vi "Geometric Match2.vi"(0 "Template File Path":path=path "C:/Users/Admin/Desktop/Main_Module_Assembly/Pattern recognition/templates/color.png", 1 "Image Src":T1, 2 "error in (no error)":errorcluster, 3 "Minimum Match Score":sgl=800.0) -> (4 "Score":dbl, 5 "x rel move":dbl, 6 "y rel move":dbl, 7 "Matched?":bool, 8 "error out":errorcluster)   [LabVIEW 2011]
uses:
  <vilib>/vision/Pattern Matching.llb/IMAQ GM Match Report.ctl
  <vilib>/vision/Image Controls.llb/IMAQ Image.ctl
  <vilib>/vision/NI_Vision_Development_Module.lvlib
panel:
  in  "Scale Factor":sgl=0.000429
  out "y":sgl
  out "x":sgl
  in  "ROI Descriptor":T2 {"Contours"."Type" items=["No Selection", "Point", "Line", "Rectangle", "Oval", "Polygon", "Freehand Region", "Annulus", "Unused2", "Unused3", "Broken Line", "Freehand Line", "Rotated Rectangle"]}
  in  "Color Plane":i32(ring)=5 items=["Red", "Green", "Blue", "Hue", "Saturation", "Luminance", "Value", "Intensity"]
  out "Image Out":T1(plugin-control)
  out "Calibrated Matches (Geometric Matching 1)":T3[](array[typedef]) {"Correlation Score" format="%.2f"; "Target Template Curve Score" format="%.2f"; "Template Target Curve Score" format="%.2f"; "Bounding Box"."y" format="%.2f"; "Bounding Box"."x" format="%.2f"; "Position"."y" format="%.2f"; "Position"."x" format="%.2f"; "Score" format="%.2f"; "Scale" format="%.2f"; "Angle" format="%.2f"; "Occlusion %" format="%.2f"}
  out "Number of Matches (Geometric Matching 1)":i32
  out "Matches (Geometric Matching 1)":T3[](array[typedef]) {"Correlation Score" format="%.2f"; "Target Template Curve Score" format="%.2f"; "Template Target Curve Score" format="%.2f"; "Bounding Box"."y" format="%.2f"; "Bounding Box"."x" format="%.2f"; "Position"."y" format="%.2f"; "Position"."x" format="%.2f"; "Score" format="%.2f"; "Scale" format="%.2f"; "Angle" format="%.2f"; "Occlusion %" format="%.2f"}
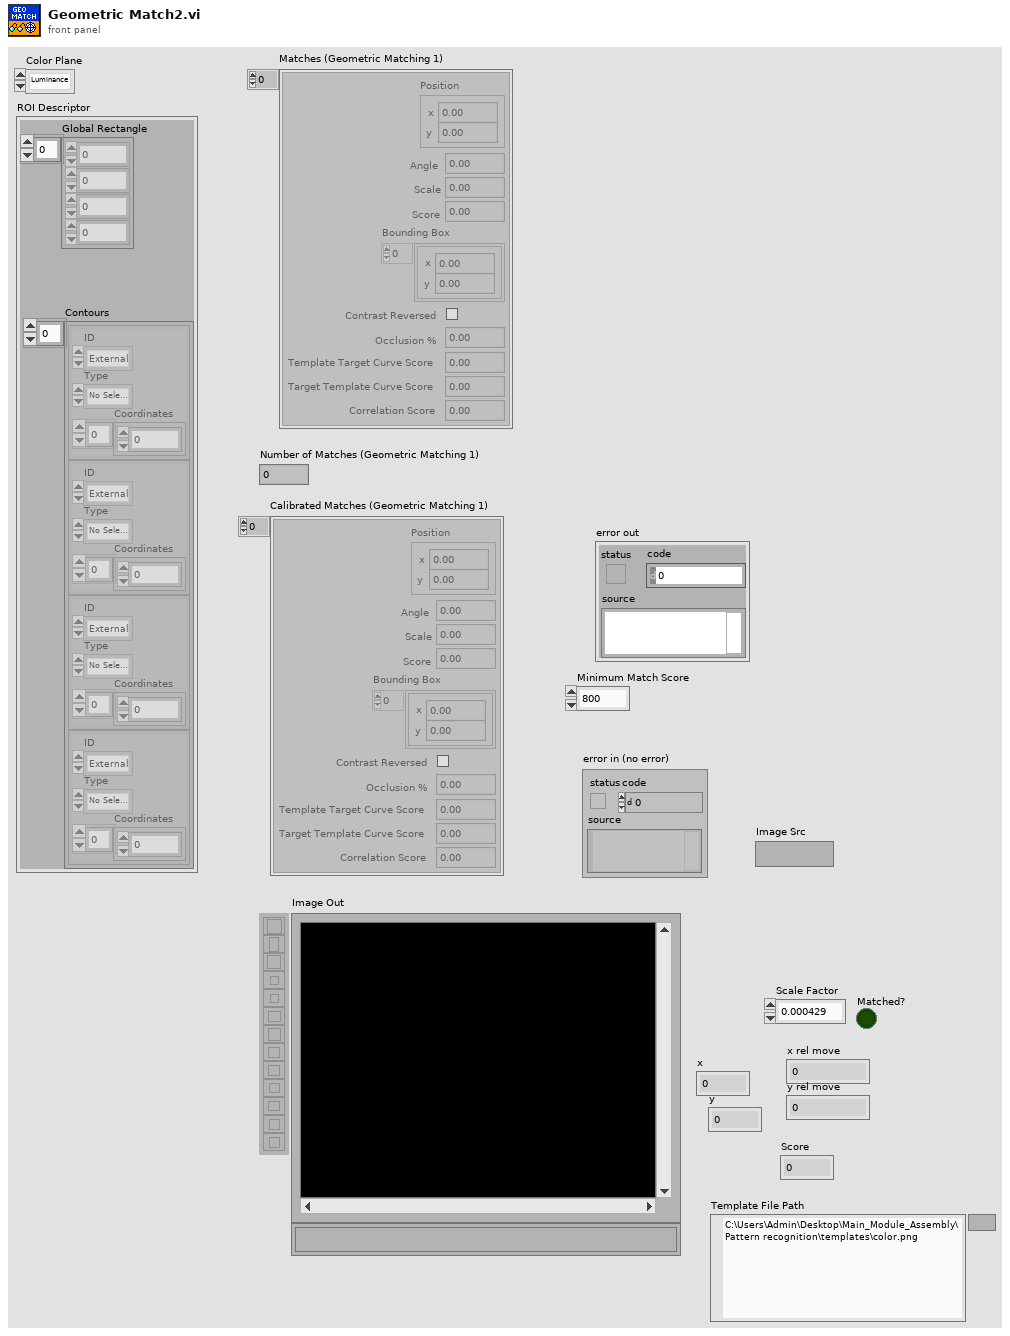
[diagram p1: front panel]
types:
  T1 = typedef "IMAQ Image.ctl" = refnum<image>
  T2 = cluster{"Global Rectangle":i32[], "Contours":cluster{"ID":enum32{"External", "Internal"}, "Type":u32, "Coordinates":i32[]}[]}
  T3 = typedef "IMAQ GM Match Report.ctl" = cluster{"Position":cluster{"x":sgl, "y":sgl}, "Angle":sgl, "Scale":sgl, "Score":sgl, "Bounding Box":cluster{"x":sgl, "y":sgl}[], "Contrast Reversed":bool, "Occlusion %":sgl, "Template Target Curve Score":sgl, "Target Template Curve Score":sgl, "Correlation Score":sgl}
  T4 = cluster{"Setup Data Item":u16, "Item Value":dbl}[]
  T5 = cluster{"Match Constraints":u32, "Min":dbl, "Max":dbl}[]
  T6 = cluster{"Rotation":bool, "Scale":bool, "Occlusion":bool, "Reserved":bool, "Reserved":bool, "Reserved":bool}
  T7 = cluster{"Extraction Mode":u32, "Edge Threshold":i32, "Edge Filter Size":u32, "Min Length":i32, "Row Search Step Size":i32, "Col Search Step Size":i32, "Max Endpoint Gap":i32, "Closed":bool, "Subpixel":bool}
  T8 = cluster{"Curve Parameters":cluster{"Extraction Mode":u32, "Edge Threshold":i32, "Edge Filter Size":u32, "Min Length":i32, "Row Search Step Size":i32, "Col Search Step Size":i32, "Max Endpoint Gap":i32, "Closed":bool, "Subpixel":bool}, "Match Mode":cluster{"Rotation":bool, "Scale":bool, "Occlusion":bool, "Reserved":bool, "Reserved":bool, "Reserved":bool}, "Range Settings":cluster{"Match Constraints":u32, "Min":dbl, "Max":dbl}[], "Number of Matches Requested":i32, "Minimum Match Score":sgl, "Subpixel Accuracy":bool, "Advanced Geometric Match Options":cluster{"Setup Data Item":u16, "Item Value":dbl}[]}
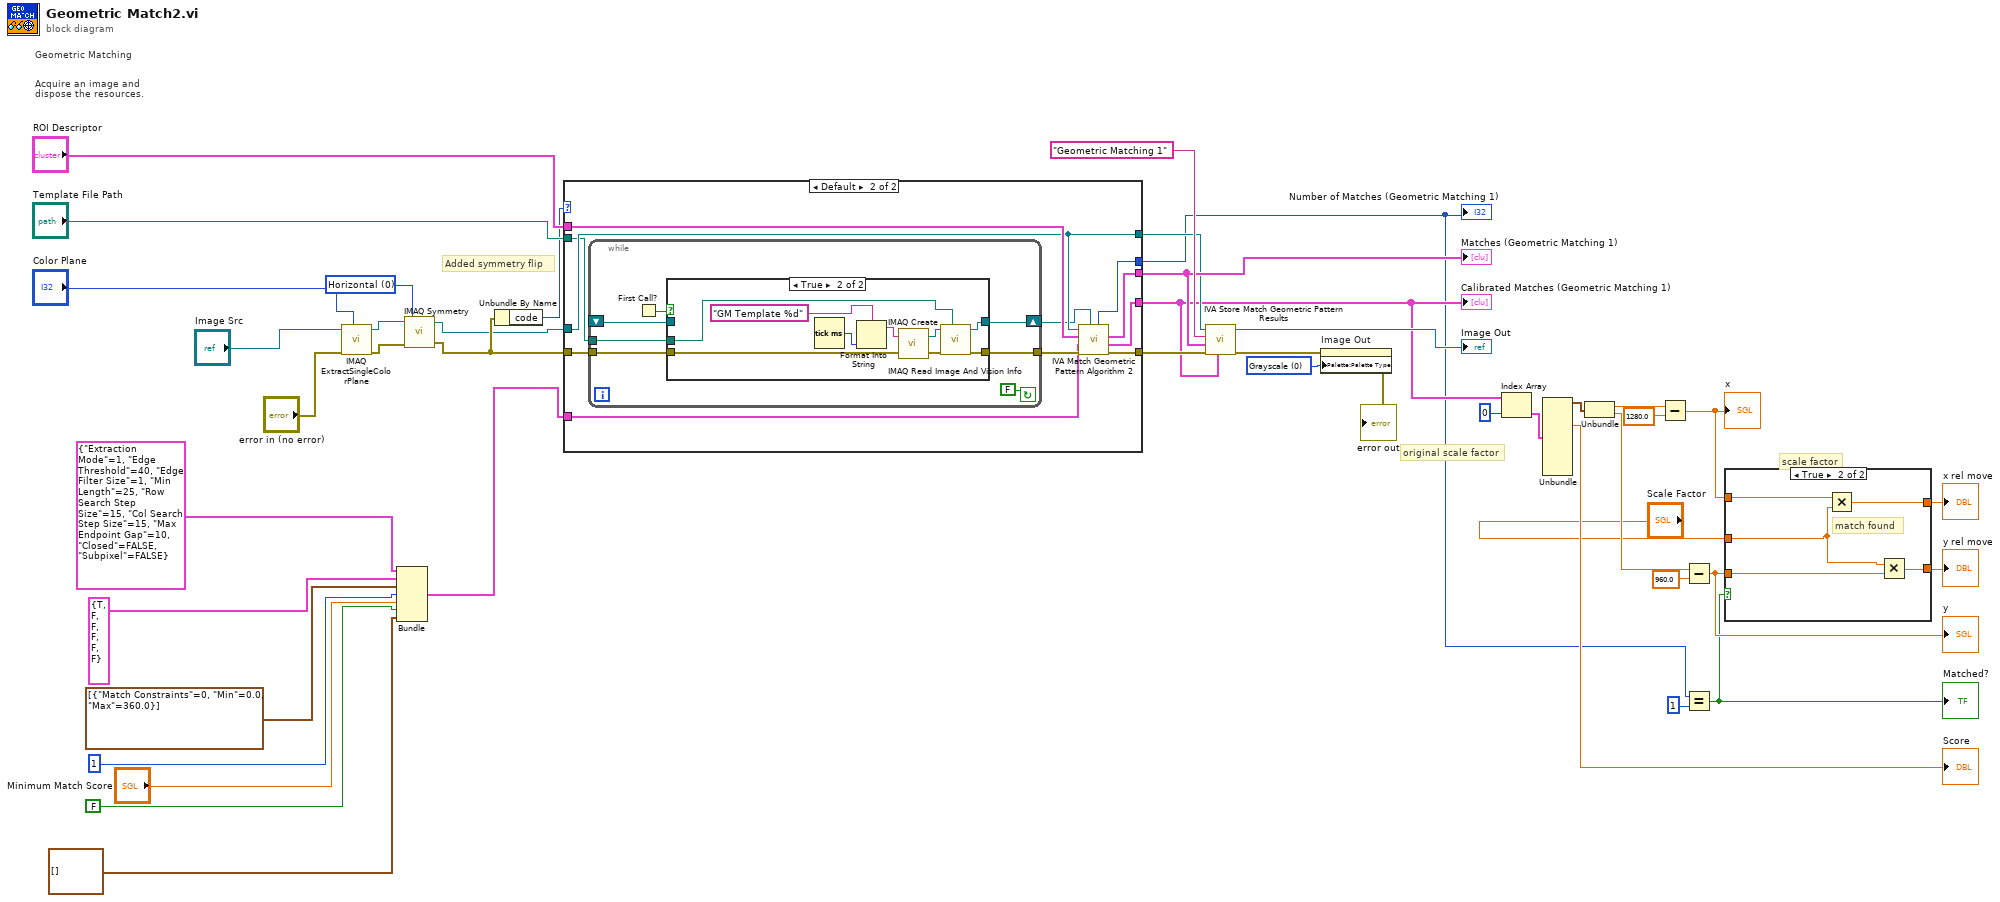
[diagram p0: block diagram]
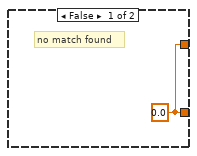
[diagram p2: hidden frame]
diagram:
  w3 = u32 0 items=["Horizontal", "Vertical", "Central", "1st Diagonal", "2nd Diagonal"] ("Type of Symmetry")
  w34 = u32 0 items=["Grayscale", "Binary", "Gradient", "Rainbow", "Temperature", "User Defined"] ("Palette")
  # "Added symmetry flip"
  # "original scale factor"
  # "scale factor"
  # "Geometric Matching"
  # "Acquire an image and\ndispose the resources."
  n1 = call "IMAQ ExtractSingleColorPlane"("Color Plane"="Color Plane", "error in (no error)"="error in (no error)", "Image Src"="Image Src") -> ("error out"=w5:errorcluster, "Image Dst Out"=w2:T1)  [unwired: 7 in]
  n2 = Bundle("Curve Parameters"=T7 {"Extraction Mode"=1, "Edge Threshold"=40, "Edge Filter Size"=1, "Min Length"=25, "Row Search Step Size"=15, "Col Search Step Size"=15, "Max Endpoint Gap"=10, "Closed"=FALSE, "Subpixel"=FALSE}, "Match Mode"=T6 {"Rotation"=TRUE, "Scale"=FALSE, "Occlusion"=FALSE, "Reserved"=FALSE, "Reserved"=FALSE, "Reserved"=FALSE}, "Range Settings"=T5 [{"Match Constraints"=0, "Min"=0.0, "Max"=360.0}], "Number of Matches Requested"=1, "Minimum Match Score"="Minimum Match Score", "Subpixel Accuracy"=FALSE, "Advanced Geometric Match Options"=T4 []) -> (w9:T8)  [unwired: 1 in]
  n3 = call "IMAQ Symmetry"("error in (no error)"=w5, "Type of Symmetry"=w3, "Image Src"=w2) -> ("error out"=w4:errorcluster, "Image Dst Out"=w1:T1)  [unwired: 2 in]
  n4 = Unbundle By Name(w4) -> ("code"=w37:i32)
  n5 = case shown="Default" w37 {
    tunnel: "Template File Path" -> [_ w50]
    tunnel: w4 -> [_ w49]
    tunnel: "ROI Descriptor" -> [_ w56]
    tunnel: w1 -> [w45 w51]
    tunnel: [_ w55] -> w41
    tunnel: [_ w54] -> w38
    tunnel: [_ w53] -> w18
    tunnel: [_ w52] -> w17
    tunnel: [w45 w51] -> w36
    tunnel: w9 -> [_ w46]
    frame -1074396199, -1074396198 {
      # "Discard Coordinate System Error"
    }
    frame Default {
      n6 = while {
        shift-right: [w62] -> w47
        shift-left: _ -> [w61]
        tunnel: [w59] -> w48
        tunnel: w49 -> [w58]
        tunnel: w50 -> [w57]
        stop <- FALSE continue-if-true
        n7 = First Call?() -> (First Call?: T/F=w63:bool)
        n8 = case shown="True" w63 {
          tunnel: [w65 w71] -> w62
          tunnel: w61 -> [w65 _]
          tunnel: [w64 w68] -> w59
          tunnel: w58 -> [w64 w67]
          tunnel: w57 -> [_ w66]
          frame False {
          }
          frame True {
            n9 = Tick Count (ms)() -> (millisecond timer value=w74:u32)
            n10 = Format Into String(format string="GM Template %d" ("Image Name"), w74) -> (resulting string=w73:string)  [unwired: 2 in, 1 out]
            n11 = call "IMAQ Create"("Image Name"=w73, "error in (no error)"=w67) -> ("New Image"=w70:T1, "error out"=w69:errorcluster)  [unwired: 3 in]
            n12 = call "IMAQ Read Image And Vision Info"("File Path"=w66, "error in (no error)"=w69, "Image"=w70) -> ("error out"=w68:errorcluster, "Image Out"=w71:T1)  [unwired: 6 in, 1 out]
          }
        }
      }
      n13 = call <vilib>:"IVA Match Geometric Pattern Algorithm 2.vi"("Template"=w47, "error in (no error)"=w48, "Settings"=w46, "ROI Descriptor"=w56, "Image"=w51) -> ("error out"=w55:errorcluster, "Calibrated Matches"=w53:T3[], "Matches"=w54:T3[], "Number of Matches"=w52:i32)  [unwired: 3 in]
    }
  }
  "Matches (Geometric Matching 1)" <- w38
  "Number of Matches (Geometric Matching 1)" <- w17
  "Calibrated Matches (Geometric Matching 1)" <- w18
  n14 = call <vilib>:"IVA Store Match Geometric Pattern Results.vi"("Calibrated Matches"=w18, "error in (no error)"=w41, "Matches"=w38, "Step Name"="Geometric Matching 1", "Image in"=w36) -> ("error out"=w40:errorcluster, "Image dup"=→"Image Out":T1)  [unwired: 5 in]
  n15 = property on="Image Out" class="ImageControl"(error in=w40, "Palette:Palette Type"=w34) -> (error out=→"error out":errorcluster)  [unwired: 1 in, 1 out]
  n16 = Index Array(array=w18, index=0) -> (element=w24:T3)
  n17 = Unbundle(w24) -> ("Position"=w21:cluster{"x":sgl, "y":sgl}, "Score"=→"Score":sgl)  [unwired: 8 out]
  n18 = Unbundle(w21) -> ("x"=w23:sgl, "y"=w22:sgl)
  n19 = Subtract(x=w23, y=sgl 1280.0) -> (x-y=w30:sgl)
  "x" <- w30
  n20 = Subtract(x=w22, y=sgl 960.0) -> (x-y=w31:sgl)
  "y" <- w31
  n21 = Equal?(x=w17, y=1) -> (x = y?=w28:bool)
  "Matched?" <- w28
  n22 = case shown="True" w28 {
    tunnel: w31 -> [_ w80]
    tunnel: w30 -> [_ w79]
    tunnel: [w75 w78] -> w27
    tunnel: [w75 w77] -> w26
    tunnel: "Scale Factor" -> [_ w76]
    frame False {
      w75 = sgl 0.0
      # "no match found"
    }
    frame True {
      # "match found"
      n23 = Multiply(x=w79, y=w76) -> (x*y=w78:sgl)
      n24 = Multiply(x=w76, y=w80) -> (x*y=w77:sgl)
    }
  }
  "x rel move" <- w27
  "y rel move" <- w26
